vi "InitializeLithographyPoints.vi"(8 "error in (no error)":errorcluster, 11 "Asylum_Driver in":refnum<class "Asylum_Driver.lvclass">) -> (0 "error out":errorcluster, 3 "Asylum_Driver out":refnum<class "Asylum_Driver.lvclass">)   [LabVIEW 2019, in "Asylum_Driver.lvclass"]
uses:
  Asylum_Driver.lvclass
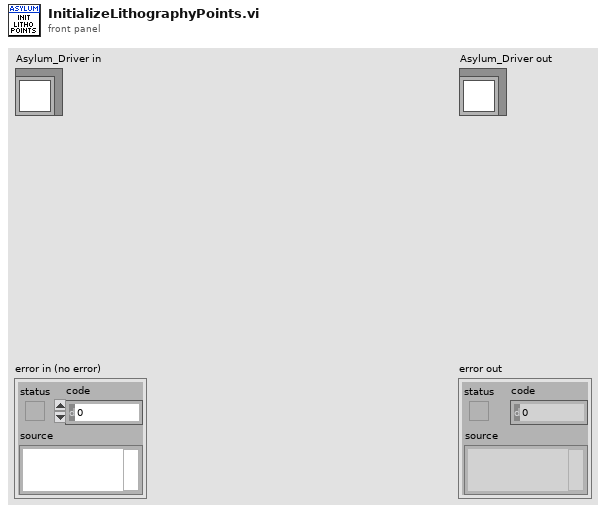
[diagram p1: front panel]
types:
  T1 = cluster{"setpoint":dbl, "pgain":dbl, "igain":dbl, "sgain":dbl}
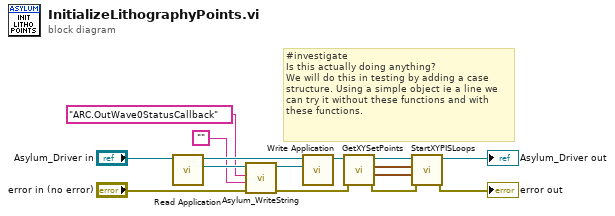
[diagram p0: block diagram]
diagram:
  # "#investigate\nIs this actually doing anything?\nWe will do this in testing by adding a case structure. Using a simple object ie a line we can try it without these functions and with these functions."
  n1 = call-dynamic "Read Application.vi"("Asylum_Driver in"="Asylum_Driver in") -> ("Application"=w14:refnum<k7>, "Asylum_Driver out"=w15:refnum<class "Asylum_Driver.lvclass">)  [unwired: 9 in]
  n2 = call <userlib>:"Asylum_WriteString.vi"("error in (no error)"="error in (no error)", "valueString"="", "parameterName"="ARC.OutWave0StatusCallback", "Application"=w14) -> ("error out"=w2:errorcluster, "Application"=w13:refnum<k7>)  [unwired: 6 in]
  n3 = call-dynamic "Write Application.vi"("Application"=w13, "Asylum_Driver in"=w15) -> ("Asylum_Driver out"=w6:refnum<class "Asylum_Driver.lvclass">)  [unwired: 9 in]
  n4 = call "GetXYSetPoints.vi"("error in (no error)"=w2, "Asylum_Driver in"=w6) -> ("error out"=w7:errorcluster, "Y PIS Controls"=w8:T1, "X PIS Controls"=w9:T1, "Asylum_Driver out"=w10:refnum<class "Asylum_Driver.lvclass">)  [unwired: 6 in]
  n5 = call "StartXYPISLoops.vi"("error in (no error)"=w7, "Y PIS Controls"=w8, "X PIS Controls"=w9, "Asylum_Driver in"=w10) -> ("error out"=→"error out":errorcluster, "Asylum_Driver out"=→"Asylum_Driver out":refnum<class "Asylum_Driver.lvclass">)  [unwired: 6 in]
